vi "Example Actor.vi"(8 "error in (no error)":errorcluster, 9 "Parent ID":string, 10 "Levels to Spawn":i32, 11 "Actors/Level":i32) -> (0 "error out":errorcluster, 3 "Example Actor out":refnum<class "Example Actor.lvclass">)   [LabVIEW 2020, in "Example Actor.lvlib" / "Example Actor.lvclass"]
doc: "Constructor to create a test actor with appropriate internal settings for the intended test."
uses:
  Example Actor.lvclass
  Example Actor.lvclass/Example Actor.ctl
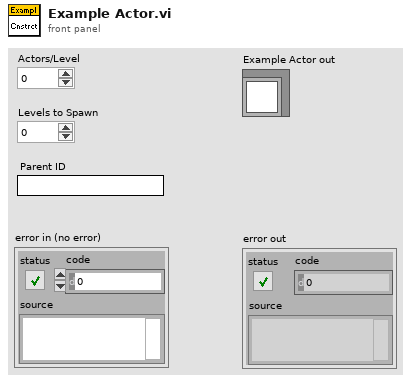
[diagram p1: front panel]
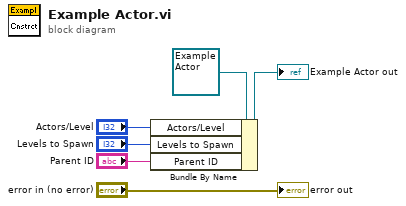
[diagram p0: block diagram]
diagram:
  n1 = Bundle By Name(cluster=refnum<class "Example Actor.lvclass"> refnum ("Test Actor.lvlib:Test Actor.lvclass"), "Actors/Level"="Actors/Level", "Levels to Spawn"="Levels to Spawn", "Parent ID"="Parent ID") -> (→"Example Actor out":refnum<class "Example Actor.lvclass">)
  "error out" <- "error in (no error)"
